vi "Get DVR from Circular Buffer.vi"(7 "Timeout in (ms)":i32=100, 8 "error in (no error)":errorcluster, 9 "Number of Waveforms":i32=2, 10 "Ignore Read Lock":bool, 11 "CIF_NIChn_FIFO_DAQ in":refnum<class "CIF_NIChn_FIFO_DAQ.lvclass">) -> (0 "error out":errorcluster, 1 "Timeout":bool, 2 "DVRs":refnum<data-value>[](array[refnum]), 3 "CIF_NIChn_FIFO_DAQ out":refnum<class "CIF_NIChn_FIFO_DAQ.lvclass">, 5 "Remaining timeout (ms)":i32=100)   [LabVIEW 2021, in "CIF_NIChn_FIFO_DAQ.lvclass"]
uses:
  CIF_NIChn_FIFO_DAQ.lvclass
  FIFO_DAQ_DVR/CIF_NIChn_FIFO_DAQ_DVR.lvclass
  D:/dev/Packages/Channel_Manager/src/CIF_NIChn/FIFO_U8/CIF_NIChn_Fifo_U8.lvclass
  D:/dev/Packages/Channel_Manager/src/CIF_NIChn/NIChn/CIF_NIChn.lvclass
  D:/dev/Packages/Channel_Manager/src/CIFChannels/CIFChannels.lvclass
  D:/dev/Packages/Channel_Manager/src/CIF_NIChn/Archive/FIFO_DAQ/CIF_NIChn_FIFO_DAQ.lvclass
  ChannelCommon/typedef/Datatype Waveform.ctl
  ChannelCommon/ChannelCommon.lvlib
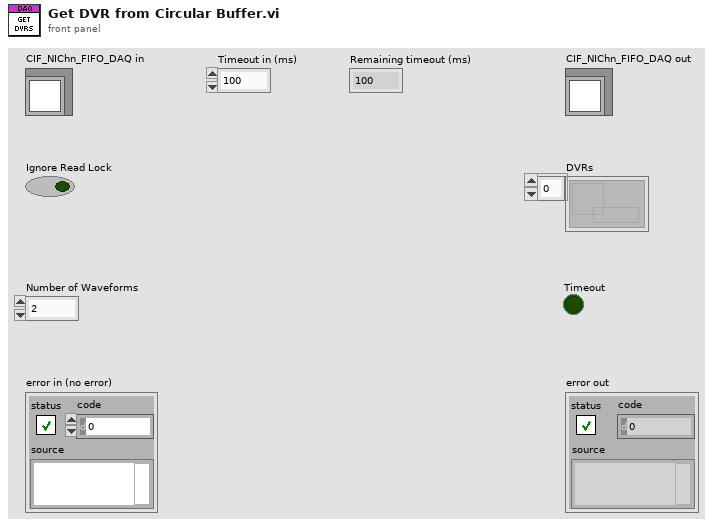
[diagram p1: front panel]
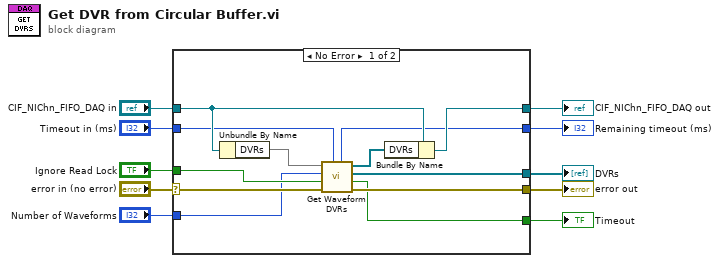
[diagram p0: block diagram]
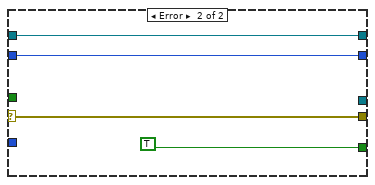
[diagram p2: hidden frame]
diagram:
  n1 = case shown="No Error" "error in (no error)" {
    selector: "error in (no error)" -> [w19 w26]
    tunnel: [w18 w26] -> w4
    tunnel: [w21 w25] -> w5
    tunnel: "CIF_NIChn_FIFO_DAQ in" -> [w22 w25]
    tunnel: "Ignore Read Lock" -> [w14 _]
    tunnel: [w16 _] -> w8
    tunnel: [w15 TRUE ("Read Lock")] -> w9
    tunnel: "Timeout in (ms)" -> [w13 w23]
    tunnel: [w12 w23] -> w6
    tunnel: "Number of Waveforms" -> [w11 _]
    frame No Error {
      n2 = Unbundle By Name(w22) -> ("DVRs"=w20)
      n3 = call "Get Waveform DVRs.vi"("Timeout in (ms)"=w13, "error in (no error)"=w19, "Ignore Read Lock"=w14, "Number of Waveforms"=w11, "DVR Circular Buffer in"=w20) -> ("error out"=w18:errorcluster, "Timeout"=w15:bool, "DVRs"=w16:refnum<data-value>[], "DVR Circular Buffer out"=w17:refnum<data-value>[], "Remaining timeout (ms)"=w12:i32)  [unwired: 2 in]
      n4 = Bundle By Name(cluster=w22, "DVRs"=w17) -> (w21:refnum<class "CIF_NIChn_FIFO_DAQ.lvclass">)
    }
    frame Error {
    }
  }
  "error out" <- w4
  "CIF_NIChn_FIFO_DAQ out" <- w5
  "Timeout" <- w9
  "DVRs" <- w8
  "Remaining timeout (ms)" <- w6
